vi "SetName.vi"(8 "Error In":errorcluster, 10 "Name":string, 11 "object in":refnum<class "YAFTAF.lvclass">) -> (0 "Error Out":errorcluster, 3 "object out":refnum<class "YAFTAF.lvclass">)   [LabVIEW 2021, in "YAFTAF.lvclass"]
uses:
  YAFTAF.lvclass
  C:/Localdata/Projects/TriekselSoft/TriekselsoftApplicationFramework/Source/.Externals/Library_YAF/YActor/YActor.lvclass
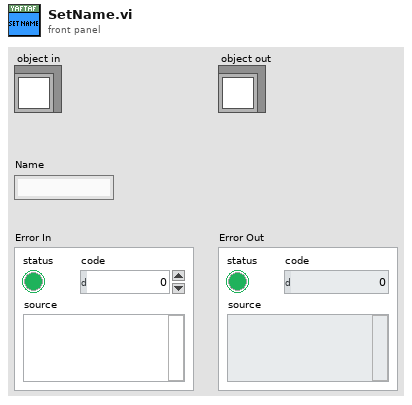
[diagram p1: front panel]
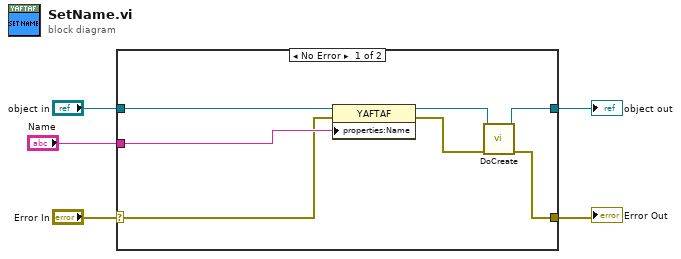
[diagram p0: block diagram]
diagram:
  n1 = case shown="No Error" "Error In" {
    selector: "Error In" -> [w10 w14]
    tunnel: [w6 w14] -> w4
    tunnel: [w8 w13] -> w2
    tunnel: "object in" -> [w12 w13]
    tunnel: "Name" -> [w11 _]
    frame No Error {
      n2 = property class="YAFTAF"(reference=w12, error in=w10, "properties:Name"=w11) -> (reference out=w9:refnum<class "YAFTAF.lvclass">, error out=w7:errorcluster)
      n3 = call-dynamic "DoCreate.vi"("ErrorIn"=w7, "ReferenceIn"=w9) -> ("ErrorOut"=w6:errorcluster, "ReferenceOut"=w8:refnum<class "YAFTAF.lvclass">)  [unwired: 8 in]
    }
    frame Error {
    }
  }
  "Error Out" <- w4
  "object out" <- w2
